vi "Sorted Particle Report Port.vi"(8 "Min Area Size %":dbl, 9 "Particle Count Limit":i32=2147483647, 10 "Pixel Measurements":T2[](array[typedef])=[35, 4, 5, 6, 7] items=["Center of Mass X", "Center of Mass Y", "First Pixel X", "First Pixel Y", "Bounding Rect Left", "Bounding Rect Top", "Bounding Rect Right", "Bounding Rect Bottom", "Max Feret Diameter Start X", "Max Feret Diameter Start Y", "Max Feret Diameter End X", "Max Feret Diameter End Y", "Max Horiz. Segment Length Left", "Max Horiz. Segment Length Right", "Max Horiz. Segment Length Row", "-", "Bounding Rect Width", "Bounding Rect Height", "Bounding Rect Diagonal", "Perimeter", "Convex Hull Perimeter", "Holes' Perimeter", "Max Feret Diameter", "Equivalent Ellipse Major Axis", "Equivalent Ellipse Minor Axis", "Equivalent Ellipse Minor Axis (Feret)", "Equivalent Rect Long Side", "Equivalent Rect Short Side", "Equivalent Rect Diagonal", "Equivalent Rect Short Side (Feret)", "Average Horiz. Segment Length", "Average Vert. Segment Length", "Hydraulic Radius", "Waddel Disk Diameter", "-", "Area", "Holes' Area", "Particle & Holes' Area", "Convex Hull Area", "Image Area", "-", "Number of Holes", "Number of Horiz. Segments", "Number of Vert. Segments", "-", "Orientation", "Max Feret Diameter Orientation", "-", "% Area/Image Area", "% Area/(Particle & Holes' Area)", "Ratio of Equivalent Ellipse Axes", "Ratio of Equivalent Rect Sides", "-", "Elongation Factor", "Compactness Factor", "Heywood Circularity Factor", "Type Factor", "-", "Sum X", "Sum Y", "Sum XX", "Sum XY", "Sum YY", "Sum XXX", "Sum XXY", "Sum XYY", "Sum YYY", "-", "Moment of Inertia XX", "Moment of Inertia XY", "Moment of Inertia YY", "Moment of Inertia XXX", "Moment of Inertia XXY", "Moment of Inertia XYY", "Moment of Inertia YYY", "Norm. Moment of Inertia XX", "Norm. Moment of Inertia XY", "Norm. Moment of Inertia YY", "Norm. Moment of Inertia XXX", "Norm. Moment of Inertia XXY", "Norm. Moment of Inertia XYY", "Norm. Moment of Inertia YYY", "Hu Moment 1", "Hu Moment 2", "Hu Moment 3", "Hu Moment 4", "Hu Moment 5", "Hu Moment 6", "Hu Moment 7"], 11 "Image in":T3) -> (0 "limits":T1, 1 "Sorted Data":dbl[][](array[numeric]), 2 "Good":bool, 3 "Particles":i32)   [LabVIEW 2019]
doc: "Returns the requested measurements of a binary image sorted by the first parameter (often size), and limiting the rows in the 2D array by count and by size. Pass infinity to count to avoid a limit. Pass zero to size to avoid a limit."
uses:
  <vilib>/vision/Image Controls.llb/IMAQ Image.ctl
  <vilib>/vision/NI_Vision_Development_Module.lvlib
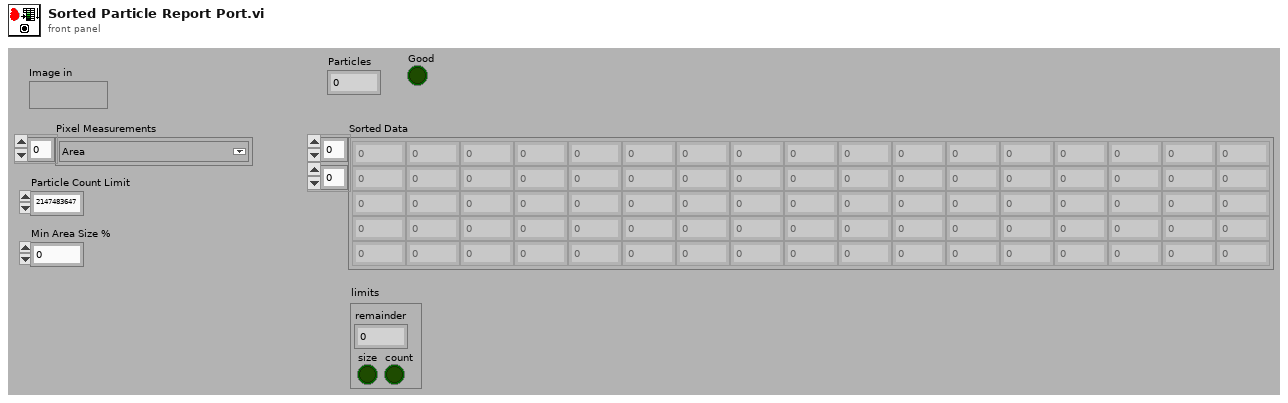
[diagram p1: front panel]
types:
  T1 = cluster{"remainder":i32, "size":bool, "count":bool}
  T2 = typedef "Particle Parameters" = i32
  T3 = typedef "IMAQ Image.ctl" = refnum<image>
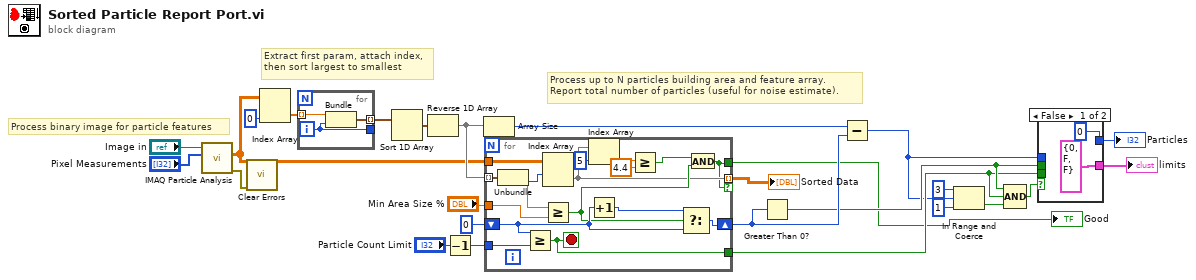
[diagram p0: block diagram]
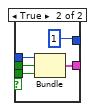
[diagram p2: hidden frame]
diagram:
  # "Process up to N particles building area and feature array.\nReport total number of particles (useful for noise estimate)."
  # "Process binary image for particle features"
  # "Extract first param, attach index,\nthen sort largest to smallest"
  n1 = call "IMAQ Particle Analysis"("Pixel Measurements"="Pixel Measurements", "Image"="Image in") -> ("error out"=w17:errorcluster, "Particle Measurements (Pixels)"=w15:dbl[][])  [unwired: 3 in, 5 out]
  n2 = call <vilib>:"Clear Errors.vi"("error in (no error)"=w17) -> ()  [unwired: 5 in, 2 out]
  n3 = Index Array(array=w15, index (col)=0 ("disabled index (col)")) -> (element=w23:dbl[])  [unwired: 1 in]
  n4 = for {
    tunnel: w23 -> [w29] mode=indexing
    tunnel: [w28] -> w24 mode=indexing
    tunnel: [w27] -> _
    i -> [w27]
    n5 = Bundle("Numeric"=w29, w27) -> (w28:cluster{"Numeric":dbl, i32})  [unwired: 1 out]
  }
  n6 = Sort 1D Array(array=w24) -> (sorted array=w25:cluster{"Numeric":dbl, i32}[])
  n7 = Reverse 1D Array(array=w25) -> (reversed array=w16:cluster{"Numeric":dbl, i32}[])
  n8 = Decrement(x="Particle Count Limit") -> (x-1=w13:i32)
  n9 = Array Size(array=w16) -> (size(s)=w19:i32)
  n10 = for {
    tunnel: w15 -> [w45]
    tunnel: w16 -> [w44] mode=indexing
    tunnel: w13 -> [w43]
    tunnel: "Min Area Size %" -> [w37]
    tunnel: [w41] -> w9
    tunnel: [w35] -> w2 mode=indexing if=w30
    shift-right: [w40] -> w11
    shift-left: 0 -> [w38]
    tunnel: [w30] -> w1
    stop <- w41 stop-if-true
    n11 = Unbundle(w44) -> ("Numeric"=w42:dbl, w46:i32)
    n12 = Greater Or Equal?(x=w38, y=w43) -> (x >= y?=w41:bool)
    n13 = Index Array(array=w45, index (row)=w46) -> (element=w35:dbl[])  [unwired: 1 in]
    n14 = Greater Or Equal?(x=w42, y=w37) -> (x >= y?=w36:bool)
    n15 = Index Array(array=w35, index=5) -> (element=w33:dbl)
    n16 = Increment(x=w38) -> (x+1=w39:i32)
    n17 = Greater Or Equal?(x=w33, y=4.4) -> (x >= y?=w31:bool)
    n18 = Select(t=w39, s=w36, f=w38) -> (s? t:f=w40:i32)
    n19 = And(x=w31, y=w36) -> (x .and. y?=w30:bool)
  }
  "Sorted Data" <- w2
  "Good" <- w1
  n20 = Greater Than 0?(x=w11) -> (x > 0?=w10:bool)
  n21 = Subtract(x=w19, y=w11) -> (x-y=w6:i32)
  n22 = In Range and Coerce(upper limit=3, x=w6, lower limit=1) -> (In Range?=w7:bool)  [unwired: 1 out]
  n23 = Compound Arithmetic op=AND(w10, w9, w7) -> (w8:bool)
  n24 = case shown="False" w8 {
    tunnel: w6 -> [_ w53]
    tunnel: [cluster{i32, bool, bool} {0, FALSE, FALSE} w52] -> w18
    tunnel: w10 -> [_ w51]
    tunnel: w9 -> [_ w50]
    tunnel: [0 1] -> w5
    frame False {
    }
    frame True {
      n25 = Bundle(w53, w51, w50) -> (w52:cluster{i32, bool, bool})  [unwired: 1 in]
    }
  }
  "Particles" <- w5
  "limits" <- w18
